vi "Auto Setup Osciloscope.vi"(8 "error in (no error)":errorcluster, 11 "EDU-X 1002A in":refnum<class "EDU-X 1002A.lvclass">) -> (0 "error out":errorcluster, 3 "EDU-X 1002A out":refnum<class "EDU-X 1002A.lvclass">)   [LabVIEW 2020, in "EDU-X 1002A.lvclass"]
uses:
  EDU-X 1002A.lvclass
  EDU-X 1002A.lvclass/EDU-X 1002A.ctl
  <instrlib>/Agilent 2000 3000 X-Series/Agilent 2000 3000 X-Series.lvlib
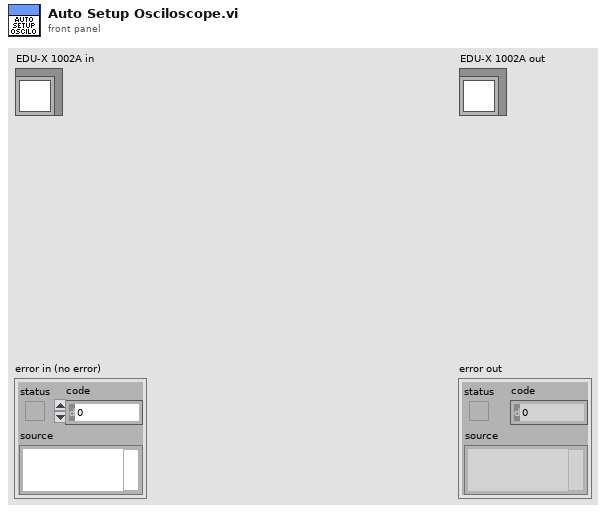
[diagram p1: front panel]
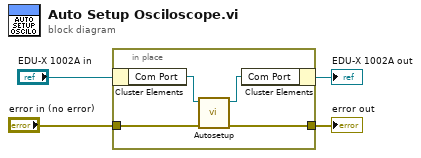
[diagram p0: block diagram]
diagram:
  n1 = in-place {
    in-place-border: "error in (no error)" -> [w6]
    in-place-border: [w5] -> w1
    n2 = in-place-cluster #1("EDU-X 1002A in") -> ("Com Port"=w8:refnum<visa-resource-name>)
    n3 = call <instrlib>:"Autosetup.vi"("error in (no error)"=w6, "VISA resource name"=w8) -> ("error out"=w5:errorcluster, "VISA resource name out"=w7:refnum<visa-resource-name>)  [unwired: 8 in]
    n4 = in-place-cluster #1("Com Port"=w7) -> (→"EDU-X 1002A out":refnum<class "EDU-X 1002A.lvclass">)
  }
  "error out" <- w1
